vi "FPGA_FGV.vi"(0 "RIO resource":T1="RIO0", 1 "Action":T2, 5 "bitfile to cache":refnum<k20>, 11 "error in":errorcluster, 12 "bus instance":u32) -> (4 "session out":refnum<class "niInstr FIFO Register Bus v1 Host.lvclass">, 6 "bitfile":refnum<k20>, 15 "error out":errorcluster)   [LabVIEW 2017]
uses:
  FPGA_FGV_action.ctl
  <vilib>/userdefined/High Color/nirio_resource_hc.ctl
  <instrlib>/_niInstr/FIFO Register Bus/v1/Host/niInstr FIFO Register Bus v1 Host.lvclass
  <vilib>/NI/Tag Bus Module Framework/FPGA manager/methods.ctl
  <vilib>/NI/Tag Bus Module Framework/FPGA manager/FPGA manager.lvlib
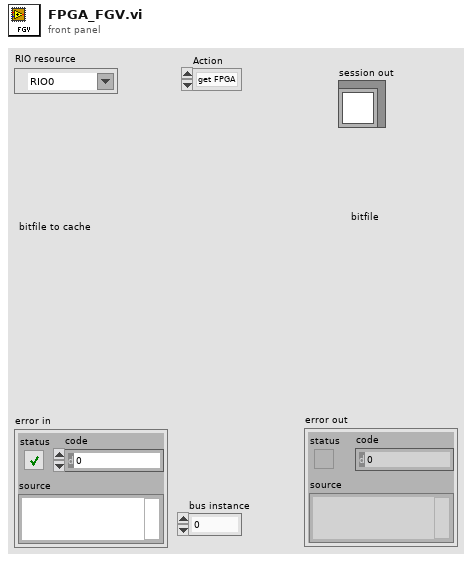
[diagram p1: front panel]
types:
  T1 = typedef "nirio_resource_hc.ctl" = tag
  T2 = typedef "FPGA_FGV_action.ctl" = enum16{"get FPGA", "set FPGA", "Close"}
  T3 = typedef "FPGA manager.lvlib/methods.ctl" = enum16{"initialize bitfile", "cache bitfile", "locate bitfile", "close bitfile", "clear manager"}
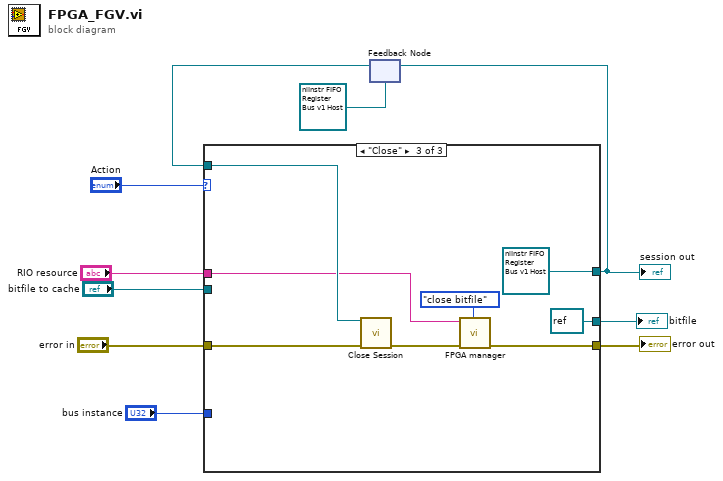
[diagram p0: block diagram]
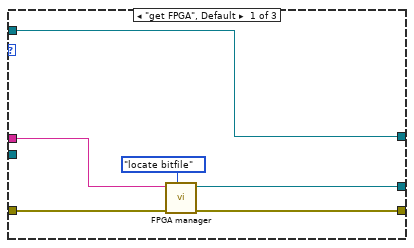
[diagram p2: hidden frame]
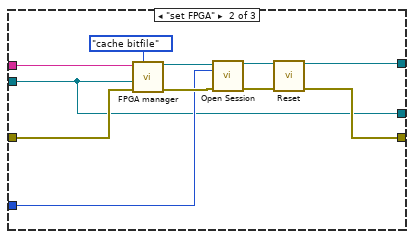
[diagram p3: hidden frame]
diagram:
  n1 = feedback #1(refnum<class "niInstr FIFO Register Bus v1 Host.lvclass"> refnum ("session out")) -> (w4:refnum<class "niInstr FIFO Register Bus v1 Host.lvclass">)
  n2 = case shown="\"Close\"" "Action" {
    tunnel: "error in" -> [w13 w22 w35]
    tunnel: [w14 w21 w30] -> w8
    tunnel: [w16 w20 refnum<class "niInstr FIFO Register Bus v1 Host.lvclass"> refnum ("session out")] -> w7
    tunnel: "RIO resource" -> [w11 w19 w29]
    tunnel: "bitfile to cache" -> [_ w17 _]
    tunnel: w4 -> [w16 _ w34]
    tunnel: [w12 w17 refnum<k20> refnum ("bitfile to cache")] -> w2
    tunnel: "bus instance" -> [_ w18 _]
    frame "get FPGA", Default {
      n3 = call <vilib>:"FPGA manager.vi"("action"=methods."locate bitfile", "error in"=w13, "RIO resource"=w11) -> ("error out"=w14:errorcluster, "bitfile"=w12:refnum<k20>)  [unwired: 6 in, 1 out]
    }
    frame "set FPGA" {
      n4 = call <vilib>:"FPGA manager.vi"("action"=methods."cache bitfile", "error in"=w22, "bitfile to cache"=w17, "RIO resource"=w19) -> ("error out"=w24:errorcluster, "bitfile"=w23:refnum<k20>)  [unwired: 5 in, 1 out]
      n5 = call <instrlib>:"Open Session.vi"("fpga ref"=w23, "bus instance"=w18, "error in"=w24) -> ("session out"=w25:refnum<class "niInstr FIFO Register Bus v1 Host.lvclass">, "error out"=w26:errorcluster)  [unwired: 11 in]
      n6 = call-dynamic "Reset.vi"("session in"=w25, "error in"=w26) -> ("session out"=w20:refnum<class "niInstr FIFO Register Bus v1 Host.lvclass">, "error out"=w21:errorcluster)  [unwired: 12 in]
    }
    frame "Close" {
      n7 = call-dynamic "Close Session.vi"("session in"=w34, "error in"=w35) -> ("error out"=w31:errorcluster)  [unwired: 13 in]
      n8 = call <vilib>:"FPGA manager.vi"("action"=methods."close bitfile", "error in"=w31, "RIO resource"=w29) -> ("error out"=w30:errorcluster)  [unwired: 6 in, 2 out]
    }
  }
  "error out" <- w8
  "session out" <- w7
  "bitfile" <- w2
  n9 = feedback-in #1(w7) -> ()
